vi "Experiment header - Update Intertrial times.vi"(8 "error in":errorcluster, 10 "Array":u64[](array[numeric]), 11 "Experiment folder path":path) -> (0 "error out":errorcluster)   [LabVIEW 2017]
panel:
  out "timings":u64[](array[numeric])
  out "Array 3":u64[](array[numeric])
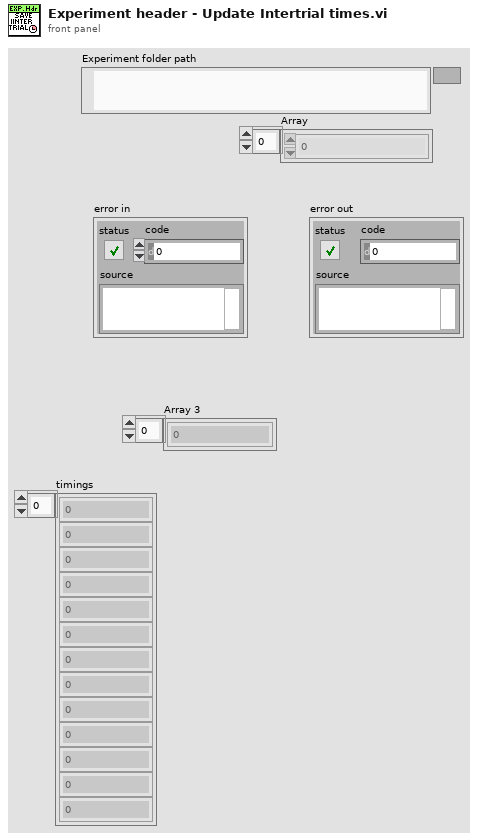
[diagram p1: front panel]
types:
  T1 = typedef "Fixed strings.ctl" = cluster{"ROI file name":string, "Normalised ROI file name":string, "Zplane Pockels values file name":string, "Functional data folder name":string, "Experiment Header file name":string, "Z-stack images folder name":string, "Groups setup rel. path":string, "Groups text file rel. path":string, "TDMS files folder name (F.img)":string, "TDMS files folder name (V.acq)":string, "TDMS files folder name (Pl.acq)":string, "Cycle rel times sequence file":string, "Dynamically called VIs folder name":string, "Time Series folder base name":string}
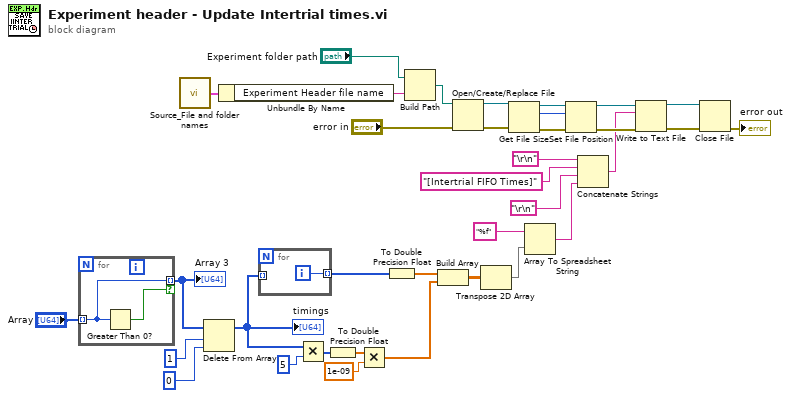
[diagram p0: block diagram]
diagram:
  n1 = for {
    tunnel: "Array" -> [w37] mode=indexing
    tunnel: [w37] -> w35 mode=indexing if=w36
    n2 = Greater Than 0?(x=w37) -> (x > 0?=w36:bool)
  }
  "Array 3" <- w35
  n3 = call "Source_File and folder names.vi"() -> ("Fixed strings"=w23:T1)  [unwired: 1 in]
  n4 = Delete From Array(array=w35, length=1, index=0) -> (array with subset deleted=w2:u64[])  [unwired: 1 out]
  "timings" <- w2
  n5 = Unbundle By Name(w23) -> ("Experiment Header file name"=w24:string)
  n6 = for {
    tunnel: w2 -> [_] mode=indexing
    tunnel: [w38] -> w1 mode=indexing
    i -> [w38]
  }
  n7 = Multiply(x=w2, y=u64 5) -> (x*y=w30:u64[])
  n8 = To Double Precision Float(number=w30) -> (double precision float=w29:dbl[])
  n9 = Multiply(x=w29, y=1e-09) -> (x*y=w27:dbl[])
  n10 = To Double Precision Float(number=w1) -> (double precision float=w26:dbl[])
  n11 = Build Path(base path="Experiment folder path", name or relative path=w24) -> (appended path=w21:path)
  n12 = Build Array(w26, w27) -> (w25:dbl[][])
  n13 = Open/Create/Replace File(file path (use dialog)=w21, error in="error in") -> (refnum out=w18:refnum<file>, error out=w19:errorcluster)  [unwired: 4 in, 1 out]
  n14 = Transpose 2D Array(2D array=w25) -> (transposed array=w3:dbl[][])
  n15 = Get File Size(file=w18, error in=w19) -> (refnum out=w17:refnum<file>, size (in bytes)=w15:i64, 0:w16:errorcluster)
  n16 = Array To Spreadsheet String(array=w3, 3:"%f" ("format string")) -> (spreadsheet string=w7:string)  [unwired: 1 in]
  n17 = Set File Position(offset (in bytes) (0)=w15, refnum=w17, error in=w16) -> (refnum out=w13:refnum<file>, error out=w14:errorcluster)  [unwired: 1 in]
  n18 = Concatenate Strings("\r\n", "[Intertrial FIFO Times]", "\r\n", w7) -> (w9:string)
  n19 = Write to Text File(file (use dialog)=w13, text=w9, error in=w14) -> (refnum out=w5:refnum<file>, error out=w6:errorcluster)  [unwired: 1 in, 1 out]
  n20 = Close File(refnum=w5, error in=w6) -> (error out=→"error out":errorcluster)  [unwired: 1 out]
